vi "Demo.vi"() -> ()   [LabVIEW 2020]
uses:
  System.Windows.Forms
  SvgDotNet.lvlib
panel:
  in  "resize":bool
  out "Color Box":u32(colorbox)
  out "Height":sgl
  out "Width":sgl
  in  "color":u32(colorbox)=16711680
  in  "Emf Path":path
  in  "Png Path":path
  in  "rasterHeight":i32=128
  in  "rasterWidth":i32=128
  in  "PictureBox":refnum<k24>(container)
  in  "SVG":path
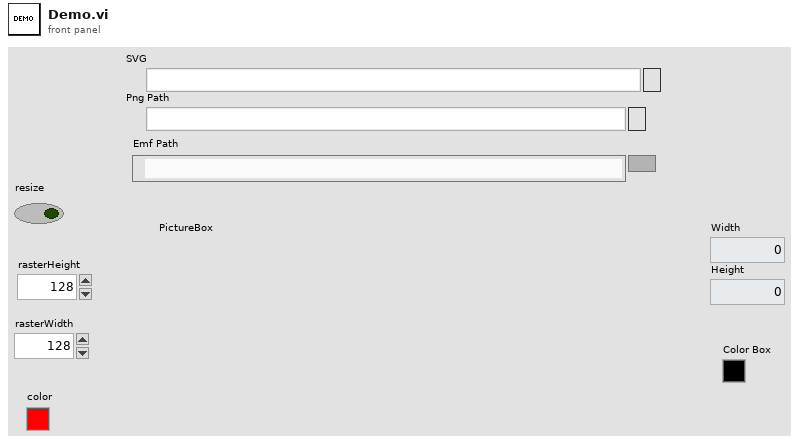
[diagram p1: front panel]
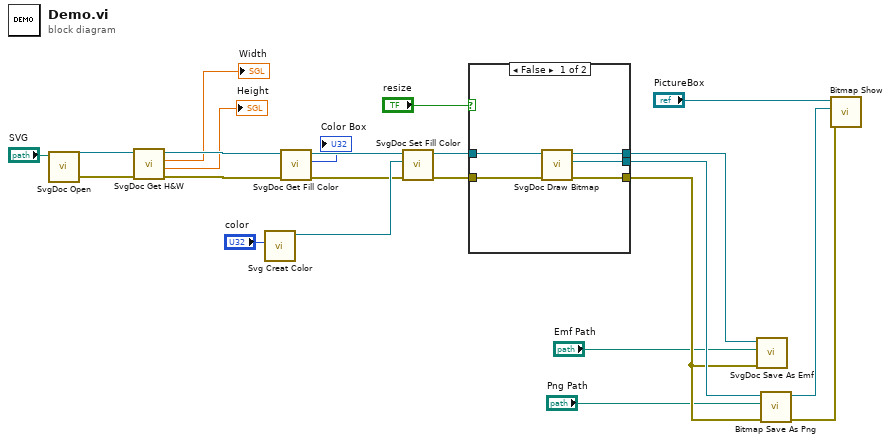
[diagram p0: block diagram]
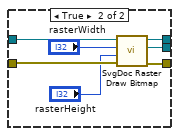
[diagram p2: hidden frame]
diagram:
  n1 = call "SvgDoc Open.vi"("SVG"="SVG") -> ("error out"=w16:errorcluster, "SVG out"=w1:refnum<k24>)  [unwired: 9 in]
  n2 = call "SvgDoc Get H&W.vi"("error in (no error)"=w16, ".NET Refnum in"=w1) -> ("error out"=w15:errorcluster, "Height"=→"Height":sgl, "Width"=→"Width":sgl, ".NET Refnum out"=w22:refnum<k24>)  [unwired: 6 in]
  n3 = call "Svg Creat Color.vi"("color"="color") -> (".NET Refnum out"=w20:refnum<k24>)  [unwired: 9 in, 1 out]
  n4 = call "SvgDoc Get Fill Color.vi"("error in (no error)"=w15, ".NET Refnum in"=w22) -> ("error out"=w14:errorcluster, "Color Box"=→"Color Box":u32, "reference out"=w21:refnum<k24>)  [unwired: 7 in]
  n5 = call "SvgDoc Set Fill Color.vi"("error in (no error)"=w14, "Color"=w20, "SVG DOC"=w21) -> ("error out"=w13:errorcluster, ".NET Refnum out"=w19:refnum<k24>)  [unwired: 7 in]
  n6 = case shown="False" "resize" {
    tunnel: w19 -> [w28 w35]
    tunnel: [w27 w34] -> w17
    tunnel: w13 -> [w24 w33]
    tunnel: [w26 w32] -> w12
    tunnel: [w25 w31] -> w10
    frame False {
      n7 = call "SvgDoc Draw Bitmap.vi"("error in (no error)"=w24, "SVG DOC"=w28) -> ("error out"=w25:errorcluster, "Bitmap"=w26:refnum<k24>, "reference out"=w27:refnum<k24>)  [unwired: 7 in]
    }
    frame True {
      n8 = call "SvgDoc Raster Draw Bitmap.vi"("error in (no error)"=w33, "rasterHeight"="rasterHeight", "rasterWidth"="rasterWidth", ".NET Refnum in"=w35) -> ("error out"=w31:errorcluster, "Bitmap"=w32:refnum<k24>, "reference out"=w34:refnum<k24>)  [unwired: 5 in]
    }
  }
  n9 = call "SvgDoc Save As Emf.vi"("error in (no error)"=w10, "Emf Path"="Emf Path", "SVG DOC"=w17) -> ()  [unwired: 7 in, 2 out]
  n10 = call "Bitmap Save As Png.vi"("error in (no error)"=w10, "Png Path"="Png Path", "Bitmap"=w12) -> ("error out"=w9:errorcluster, "Bitmap out"=w11:refnum<k24>)  [unwired: 7 in]
  n11 = call "Bitmap Show.vi"("error in (no error)"=w9, "Bitmap"=w11, "PictureBox"="PictureBox") -> ()  [unwired: 6 in, 3 out]
